vi "Modbus Multi-Read STR.vi"(7 "Slave Address":u8, 8 "error in (no error)":errorcluster, 9 "Number of chars to read\n/ length of string":i32 format="%x", 10 "Register Start Address":u16 format="%x", 11 "VISA resource in":refnum<visa-resource-name>) -> (0 "error out":errorcluster, 1 "Output string":string, 3 "VISA resource out":refnum<visa-resource-name>)   [LabVIEW 2010, in "Voegtlin_NI_SMART_Modbus_Drivers.lvlib"]
doc: "Lese einen beliebig langen String ab der angegebenen Startadresse des selektierten Geraetes aus.\nDer COM-Port muss dazu initialisiert sein (benutze\" Modbus Init.vi\")."
uses:
  Voegtlin_NI_SMART_Modbus_Drivers.lvlib
  Enums/Modbus Comm.ctl
panel:
  out "Outputdata U8 (array)":u8[](array[numeric])
  out "Read register data\n U16 (array)":u16[](array[numeric])
  # "Internal Data"
  # "Output Data"
  # "Input Data"
  # "(Inputmaske in HEX)"
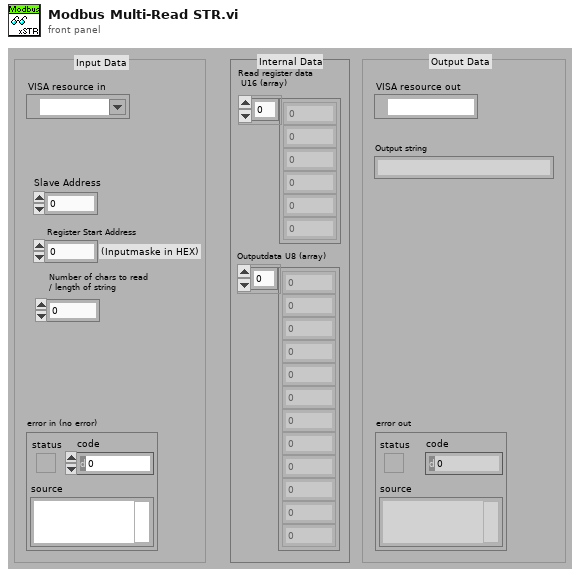
[diagram p1: front panel]
types:
  T1 = typedef "Voegtlin_NI_SMART_Modbus_Drivers.lvlib/Modbus Comm.ctl" = enum16{"Init", "Read", "Write", "Exit"}
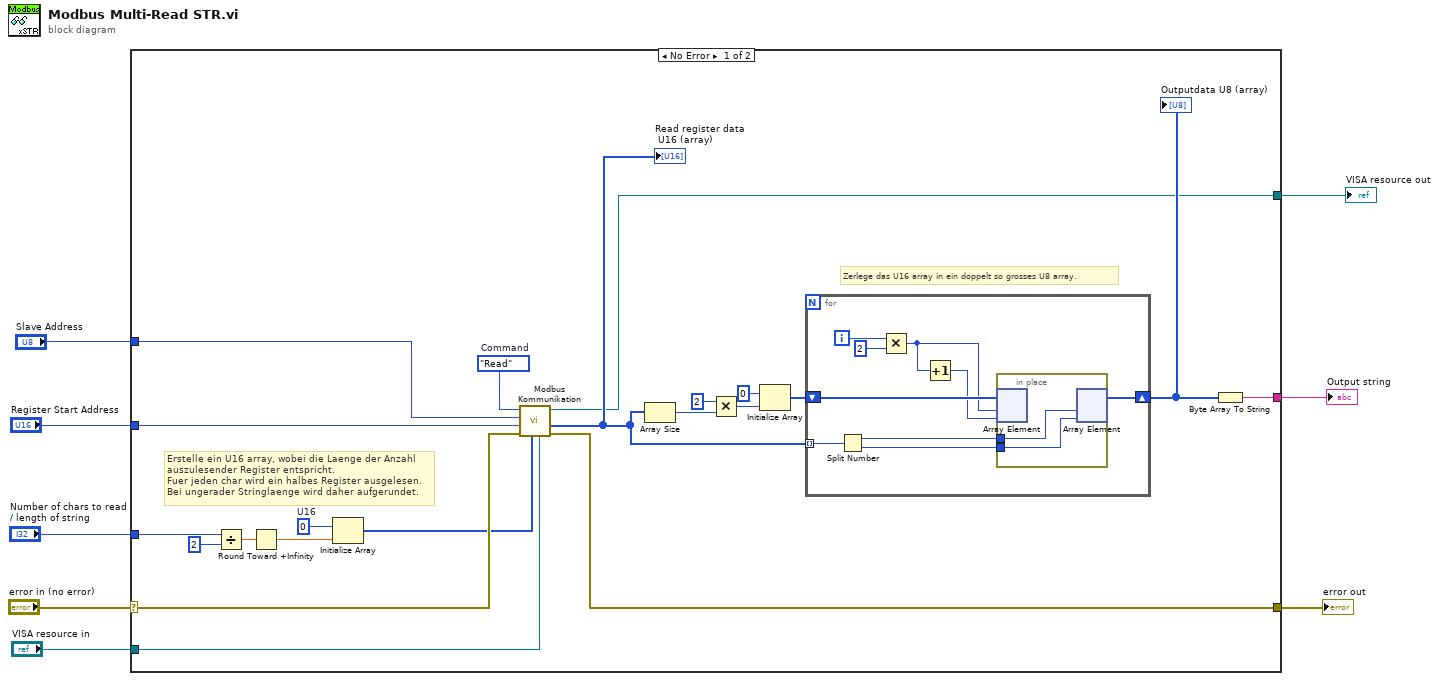
[diagram p0: block diagram]
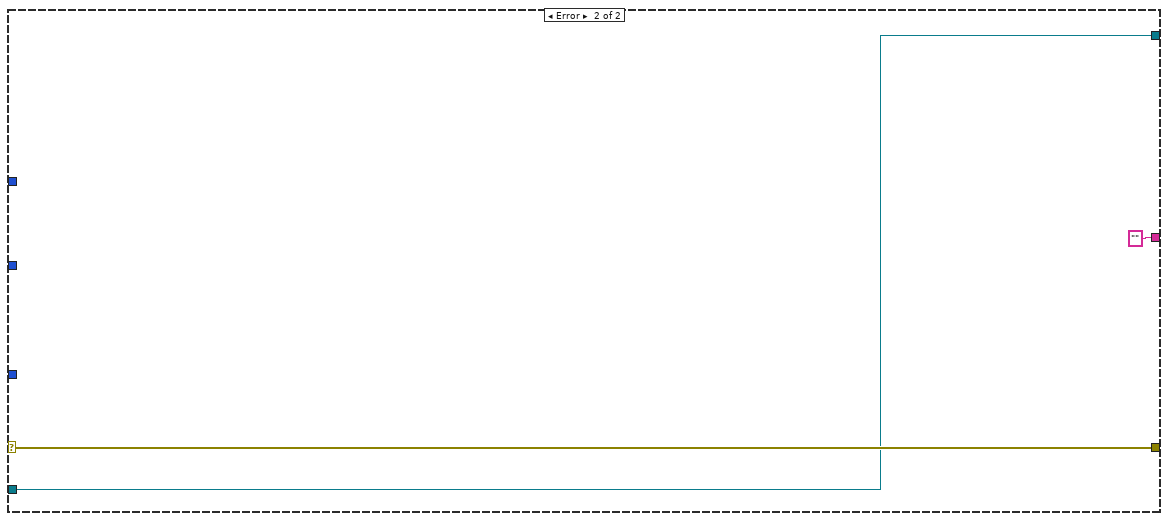
[diagram p2: hidden frame]
diagram:
  n1 = case shown="No Error" "error in (no error)" {
    selector: "error in (no error)" -> [w14 w43]
    tunnel: "Register Start Address" -> [w12 _]
    tunnel: [w29 w43] -> w7
    tunnel: "Number of chars to read\n/ length of string" -> [w26 _]
    tunnel: [w16 "" ("string")] -> w5
    tunnel: "Slave Address" -> [w11 _]
    tunnel: "VISA resource in" -> [w10 w41]
    tunnel: [w9 w41] -> w1
    frame No Error {
      w27 = u16 0  # U16
      w28 = Modbus_Comm."Read"  # Command
      # "Zerlege das U16 array in ein doppelt so grosses U8 array."
      # "Erstelle ein U16 array, wobei die Laenge der Anzahl auszulesender Register entspricht.\nFuer jeden char wird ein halbes Register ausgelesen. Bei ungerader Stringlaenge wird daher aufgerundet."
      n2 = Divide(x=w26, y=2) -> (x/y=w24:dbl)
      n3 = Round Toward +Infinity(x=w24) -> (ceil(x): smallest int >= x=w23:dbl)
      n4 = Initialize Array(w27, w23) -> (w13:u16[])
      n5 = call "Modbus Kommunikation.vi"("VISA resource in"=w10, "Data In / #Reads [U16]"=w13, "error in (no error)"=w14, "Register Start Address"=w12, "Slave Address"=w11, "Command"=w28) -> ("error out"=w29:errorcluster, "Data Out [U16]"=w17:u16[], "VISA resource out"=w9:refnum<visa-resource-name>)  [unwired: 3 in]
      "Read register data\n U16 (array)" <- w17
      n6 = Array Size(array=w17) -> (size(s)=w22:i32)
      n7 = Multiply(x=2, y=w22) -> (x*y=w20:i32)
      n8 = Initialize Array(u8 0 ("x"), w20) -> (w18:u8[])
      n9 = for {
        tunnel: w17 -> [w38] mode=indexing
        shift-right: [w30] -> w15
        shift-left: w18 -> [w35]
        i -> [w37]
        n10 = Split Number(x=w38) -> (hi(x)=w32:u8, lo(x)=w31:u8)
        n11 = Multiply(x=w37, y=2) -> (x*y=w34:i32)
        n12 = Increment(x=w34) -> (x+1=w33:i32)
        n13 = in-place {
          in-place-border: w32 -> [w40]
          in-place-border: w31 -> [w39]
          n14 = in-place-array #1(w35, w34, w33) -> ()  [unwired: 2 out]
          n15 = in-place-array #1(w40, w39) -> (w30:u8[])  [unwired: 2 out]
        }
      }
      "Outputdata U8 (array)" <- w15
      n16 = Byte Array To String(unsigned byte array=w15) -> (string=w16:string)
    }
    frame Error {
    }
  }
  "error out" <- w7
  "Output string" <- w5
  "VISA resource out" <- w1
